vi "Hide Animated Busy Icon with Message.vi"(4 "Animated Busy Icon Control Name (Animated Busy Icon)":string="Animated Busy Icon", 5 "Already active? (F)":bool, 6 "Message Control Name (Message)":string="Message", 7 "Message":string, 9 "Error In":errorcluster, 11 "Target VI reference":refnum<vi>) -> (1 "Error Out":errorcluster)   [LabVIEW 2021]
doc: "This VI passes error in through and ignores it."
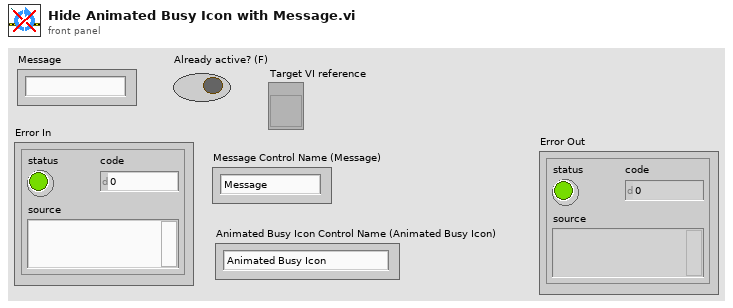
[diagram p1: front panel]
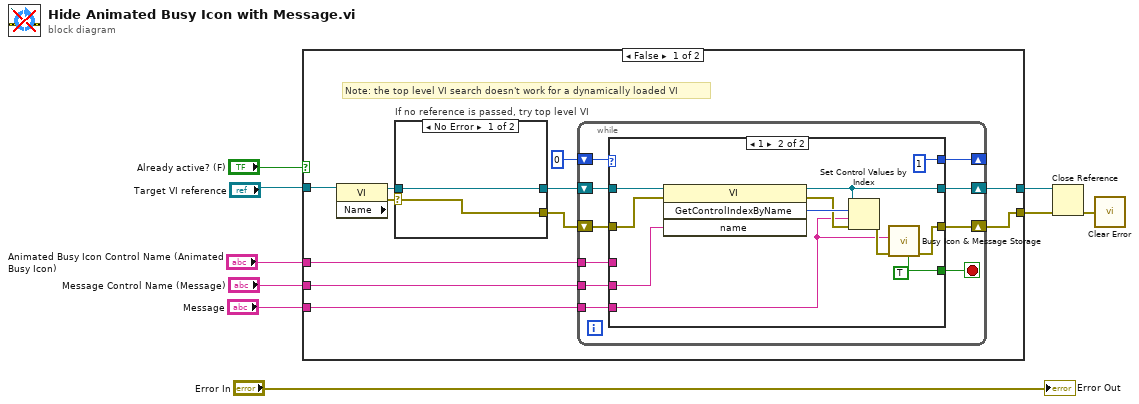
[diagram p0: block diagram]
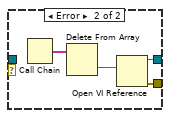
[diagram p2: hidden frame]
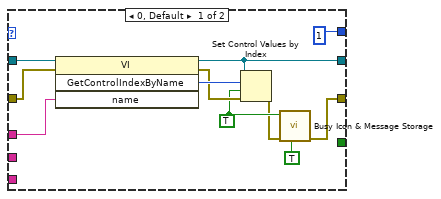
[diagram p3: hidden frame]
diagram:
  n1 = case shown="False" "Already active? (F)" {
    tunnel: [w20 w59] -> w9
    tunnel: [w19 _] -> w8
    tunnel: "Message Control Name (Message)" -> [w17 _]
    tunnel: "Animated Busy Icon Control Name (Animated Busy Icon)" -> [w16 _]
    tunnel: "Message" -> [w15 _]
    tunnel: "Target VI reference" -> [w12 w59]
    frame False {
      # "Note: the top level VI search doesn't work for a dynamically loaded VI"
      n2 = property class="VI" props=["Name"](reference=w12) -> (reference out=w11:refnum<vi>, error out=w10:errorcluster)  [unwired: 1 in, 1 out]
      n3 = case "If no reference is passed, try top level VI" shown="No Error" w10 {
        selector: w10 -> [w21 _]
        tunnel: [w21 w26] -> w13
        tunnel: [w22 w25] -> w14
        tunnel: w11 -> [w22 _]
        frame No Error {
        }
        frame Error {
          n4 = Call Chain() -> (call chain=w23:string[])
          n5 = Delete From Array(array=w23) -> (deleted portion=w24:string)  [unwired: 2 in, 1 out]
          n6 = Open VI Reference(vi path=w24) -> (vi reference=w25:refnum<vi>, error out=w26:errorcluster)  [unwired: 5 in]
        }
      }
      n7 = while {
        shift-right: [w33] -> w19
        shift-left: w13 -> [w36]
        shift-right: [w34] -> w20
        shift-left: w14 -> [w35]
        shift-right: [w31] -> _
        shift-left: 0 -> [w32]
        tunnel: w17 -> [w29]
        tunnel: w16 -> [w28]
        tunnel: w15 -> [w27]
        stop <- w30 stop-if-true
        n8 = case shown="1" w32 {
          tunnel: w36 -> [w45 w56]
          tunnel: w35 -> [w44 w55]
          tunnel: [w43 w54] -> w34
          tunnel: [w37 w50] -> w33
          tunnel: [1 1] -> w31
          tunnel: [_ w48] -> w30
          tunnel: w29 -> [_ w52]
          tunnel: w28 -> [w41 _]
          tunnel: w27 -> [_ w49]
          frame 0, Default {
            w39 = TRUE ("Visible")
            n9 = invoke class="VI" method="GetControlIndexByName"(reference=w44, error in=w45, "name"=w41) -> (reference out=w43:refnum<vi>, error out=w46:errorcluster, "GetControlIndexByName"=w47:i32)  [unwired: 1 in, 1 out]
            n10 = Set Control Values by Index(0:w43, 1:w47, 2:w39, 3:w46) -> (11:w38:errorcluster)
            n11 = call "Busy Icon & Message Storage.vi"("Get(F)/Set Busy Icon"=TRUE, "Error In"=w38, "Busy Icon Status (F = busy)"=w39) -> ("Error Out"=w37:errorcluster)  [unwired: 6 in, 2 out]
          }
          frame 1 {
            w48 = TRUE
            n12 = invoke class="VI" method="GetControlIndexByName"(reference=w55, error in=w56, "name"=w52) -> (reference out=w54:refnum<vi>, error out=w57:errorcluster, "GetControlIndexByName"=w58:i32)  [unwired: 1 in, 1 out]
            n13 = Set Control Values by Index(0:w54, 1:w58, 2:w49, 3:w57) -> (11:w51:errorcluster)
            n14 = call "Busy Icon & Message Storage.vi"("Get(F)/Set Message"=w48, "Error In"=w51, "Message String"=w49) -> ("Error Out"=w50:errorcluster)  [unwired: 6 in, 2 out]
          }
        }
      }
    }
    frame True {
      # "Leave the hiding of the busy icon to the first caller"
    }
  }
  n15 = Close Reference(reference=w9, error in (no error)=w8) -> (error out=w1:errorcluster)
  n16 = call "Clear Error.vi"("Error In"=w1) -> ()  [unwired: 8 in, 1 out]
  "Error Out" <- "Error In"
